vi "S2C_VLFT10_Proc_LaunchFornax.vi"(8 "Error In":errorcluster, 11 "Selection":string) -> (0 "Error Out":errorcluster, 3 "Version":string)   [LabVIEW 2015]
uses:
  Fornax/VIs/PolyDriver/Typedefs/ExternalCommCommand.ctl
  Fornax/VIs/S2C_FORNAX_Proc_Globals.vi
  Fornax/VIs/PolyDriver/S2C_FORNAX_Poly_CloseFornax.vi
  Fornax/VIs/PolyDriver/S2C_FORNAX_Poly_LaunchFornax.vi
  Fornax/VIs/PolyDriver/S2C_FORNAX_Poly_OpenSocket.vi
  Fornax/VIs/PolyDriver/S2C_FORNAX_Poly_ExternalCommCommand.vi
panel:
  out "Paired?":bool
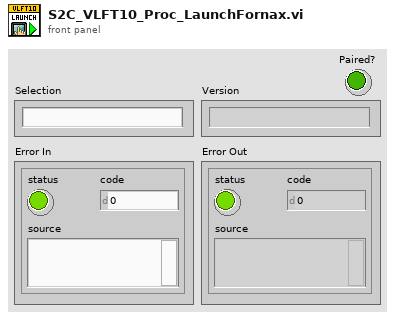
[diagram p1: front panel]
types:
  T1 = cluster{"Path":string, "Port":i32, "Version":u16}
  T2 = cluster{"Driver":string, "Command":string, "Return":string, "Parameters":string, "Timeout":dbl}
  T3 = typedef "ExternalCommCommand.ctl" = i16
  T4 = cluster{"Partition":string, "Message":string, "M_CommandOptions":string, "M_ControllerBoardId":string, "M_ClientId":string, "M_Command":T3}
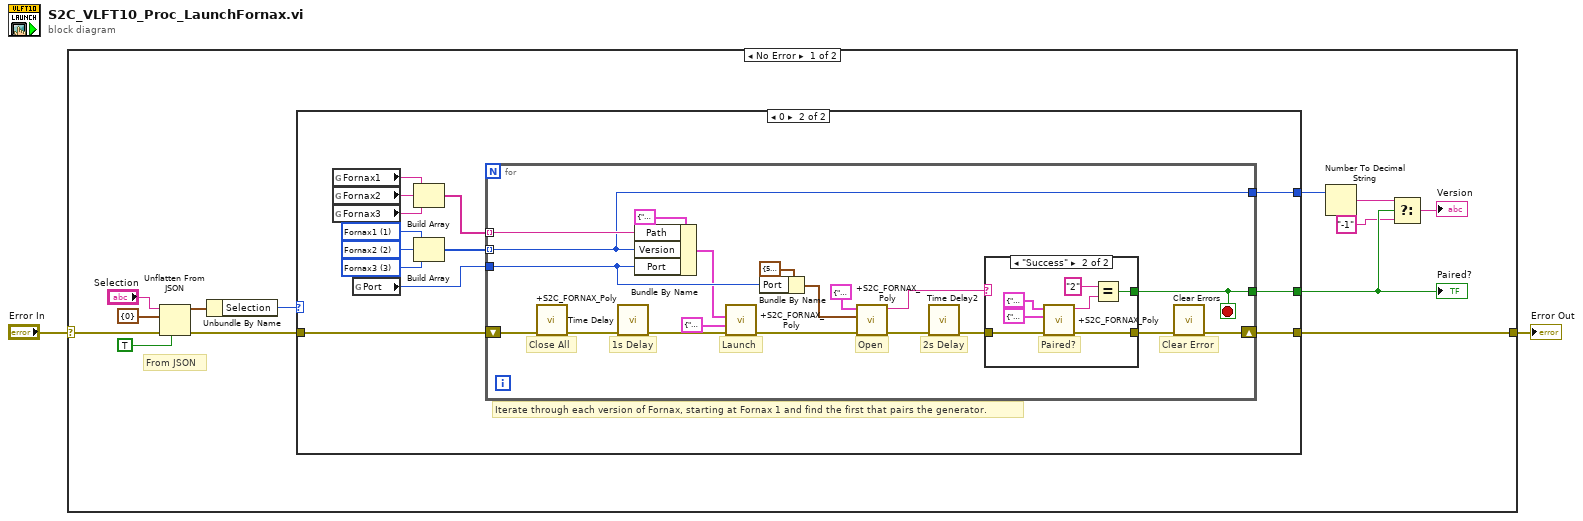
[diagram p0: block diagram]
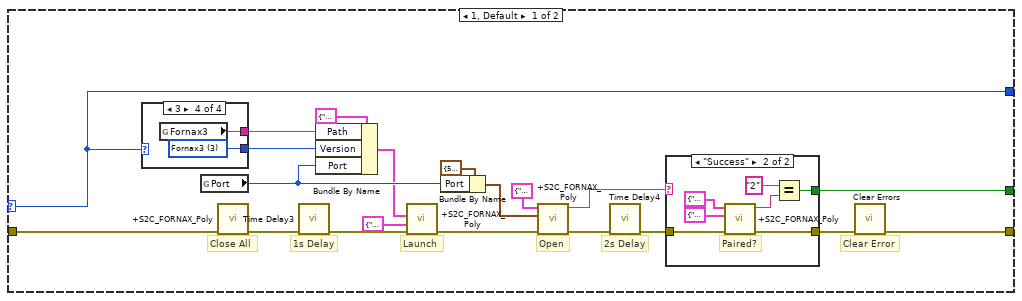
[diagram p2: hidden frame]
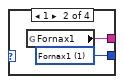
[diagram p4: hidden frame]
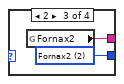
[diagram p5: hidden frame]
diagram:
  n1 = case shown="No Error" "Error In" {
    selector: "Error In" -> [w14 w90]
    tunnel: [w15 w90] -> w1
    frame No Error {
      # "From JSON"
      n2 = Unflatten From JSON(JSON string="Selection", type and defaults=cluster{"Selection":u16} {"Selection"=0}, default null elements? (F)=TRUE, error in (no error)=w14) -> (value=w9:cluster{"Selection":u16}, error out=w10:errorcluster)  [unwired: 3 in]
      n3 = Unbundle By Name(w9) -> ("Selection"=w8:u16)
      n4 = case shown="0" w8 {
        selector: w8 -> [w16 _]
        tunnel: [w34 w61] -> w15
        tunnel: [w33 w52] -> w5
        tunnel: w10 -> [w32 w51]
        tunnel: [w16 w50] -> w7
        frame 1, Default {
          # "Clear Error"
          # "2s Delay"
          # "1s Delay"
          # "Open"
          # "Launch"
          # "Close All"
          n5 = case shown="3" w16 {
            tunnel: [_ w37 w39 w41] -> w18
            tunnel: [_ w36 w38 w40] -> w17
            frame 0, Default {
            }
            frame 1 {
              w36 = u16 1 items=["Fornax1"=1, "Fornax2"=2, "Fornax3"=3] ("Version")
              n6 = global read "S2C_FORNAX_Proc_Globals.vi" "Fornax1"() -> (w37:string)
            }
            frame 2 {
              w38 = u16 2 items=["Fornax1"=1, "Fornax2"=2, "Fornax3"=3] ("Version")
              n7 = global read "S2C_FORNAX_Proc_Globals.vi" "Fornax2"() -> (w39:string)
            }
            frame 3 {
              w40 = u16 3 items=["Fornax1"=1, "Fornax2"=2, "Fornax3"=3] ("Version")
              n8 = global read "S2C_FORNAX_Proc_Globals.vi" "Fornax3"() -> (w41:string)
            }
          }
          n9 = global read "S2C_FORNAX_Proc_Globals.vi" "Port"() -> (w35:i32)
          n10 = call-poly "+S2C_FORNAX_Poly.vi"("Error In"=w32) -> ("Error Out"=w19:errorcluster)  [unwired: 9 in, 1 out]
          n11 = call "Time Delay3"("error in (no error)"=w19) -> ("error out"=w25:errorcluster)  [unwired: 10 in]
          n12 = Bundle By Name(cluster=T1 {"Path"="", "Port"=50000, "Version"=1} ("Open"), "Path"=w18, "Version"=w17, "Port"=w35) -> (w23:T1)
          n13 = call-poly "+S2C_FORNAX_Poly.vi"("Error In"=w25, "Open"=w23, "Settings"=T2 {"Driver"="Fornax", "Command"="Launch", "Return"="ErrorStatus", "Parameters"="", "Timeout"=10.0}) -> ("Error Out"=w31:errorcluster)  [unwired: 7 in, 1 out]
          n14 = Bundle By Name(cluster=cluster{"Port":i32} {"Port"=50000} ("Open"), "Port"=w35) -> (w29:cluster{"Port":i32})
          n15 = call-poly "+S2C_FORNAX_Poly.vi"("Error In"=w31, "Open"=w29, "Settings"=T2 {"Driver"="Fornax", "Command"="Open", "Return"="ErrorStatus", "Parameters"="", "Timeout"=20.0}) -> ("Error Out"=w22:errorcluster, "Response"=w27:string)  [unwired: 7 in]
          n16 = call "Time Delay4"("error in (no error)"=w22) -> ("error out"=w21:errorcluster)  [unwired: 10 in]
          n17 = case shown="\"Success\"" w27 {
            tunnel: w21 -> [w42 w49]
            tunnel: [w42 w45] -> w20
            tunnel: [_ w44] -> w33
            frame "Other", Default {
            }
            frame "Success" {
              # "Paired?"
              n18 = call-poly "+S2C_FORNAX_Poly.vi"("Error In"=w49, "ExternalCommCommand"=T4 {"Partition"="Default", "Message"="ExternalCommCommand", "M_CommandOptions"="", "M_ControllerBoardId"="", "M_ClientId"="", "M_Command"=5}, "Settings"=T2 {"Driver"="Fornax", "Command"="ExternalCommCommand", "Return"="M_PairingStatus", "Parameters"="", "Timeout"=10.0}) -> ("Error Out"=w45:errorcluster, "Response"=w47:string)  [unwired: 7 in]
              n19 = Equal?(x="2", y=w47) -> (x = y?=w44:bool)
            }
          }
          n20 = call <vilib>:"Clear Errors.vi"("error in (no error)"=w20) -> ("error out"=w34:errorcluster)  [unwired: 5 in, 1 out]
        }
        frame 0 {
          w55 = u16 3 items=["Fornax1"=1, "Fornax2"=2, "Fornax3"=3] ("Version")
          w57 = u16 2 items=["Fornax1"=1, "Fornax2"=2, "Fornax3"=3] ("Version")
          w56 = u16 1 items=["Fornax1"=1, "Fornax2"=2, "Fornax3"=3] ("Version")
          # "Iterate through each version of Fornax, starting at Fornax 1 and find the first that pairs the generator."
          n21 = global read "S2C_FORNAX_Proc_Globals.vi" "Fornax1"() -> (w59:string)
          n22 = global read "S2C_FORNAX_Proc_Globals.vi" "Fornax2"() -> (w60:string)
          n23 = global read "S2C_FORNAX_Proc_Globals.vi" "Fornax3"() -> (w58:string)
          n24 = global read "S2C_FORNAX_Proc_Globals.vi" "Port"() -> (w62:i32)
          n25 = Build Array(w59, w60, w58) -> (w54:string[])
          n26 = Build Array(w56, w57, w55) -> (w53:u16[])
          n27 = for {
            tunnel: w62 -> [w79]
            tunnel: w54 -> [w71] mode=indexing
            tunnel: w53 -> [w63] mode=indexing
            shift-right: [w67] -> w61
            shift-left: w51 -> [w64]
            tunnel: [w66] -> w52
            tunnel: [w63] -> w50
            stop <- w66 stop-if-true
            # "Clear Error"
            # "2s Delay"
            # "1s Delay"
            # "Open"
            # "Launch"
            # "Close All"
            n28 = call-poly "+S2C_FORNAX_Poly.vi"("Error In"=w64) -> ("Error Out"=w65:errorcluster)  [unwired: 9 in, 1 out]
            n29 = call "Time Delay"("error in (no error)"=w65) -> ("error out"=w74:errorcluster)  [unwired: 10 in]
            n30 = Bundle By Name(cluster=T1 {"Path"="", "Port"=50000, "Version"=1} ("Open"), "Path"=w71, "Version"=w63, "Port"=w79) -> (w72:T1)
            n31 = call-poly "+S2C_FORNAX_Poly.vi"("Error In"=w74, "Open"=w72, "Settings"=T2 {"Driver"="Fornax", "Command"="Launch", "Return"="ErrorStatus", "Parameters"="", "Timeout"=10.0}) -> ("Error Out"=w81:errorcluster)  [unwired: 7 in, 1 out]
            n32 = Bundle By Name(cluster=cluster{"Port":i32} {"Port"=50000} ("Open"), "Port"=w79) -> (w78:cluster{"Port":i32})
            n33 = call-poly "+S2C_FORNAX_Poly.vi"("Error In"=w81, "Open"=w78, "Settings"=T2 {"Driver"="Fornax", "Command"="Open", "Return"="ErrorStatus", "Parameters"="", "Timeout"=20.0}) -> ("Error Out"=w70:errorcluster, "Response"=w76:string)  [unwired: 7 in]
            n34 = call "Time Delay2"("error in (no error)"=w70) -> ("error out"=w69:errorcluster)  [unwired: 10 in]
            n35 = case shown="\"Success\"" w76 {
              tunnel: w69 -> [w82 w89]
              tunnel: [w82 w85] -> w68
              tunnel: [_ w84] -> w66
              frame "Other", Default {
              }
              frame "Success" {
                # "Paired?"
                n36 = call-poly "+S2C_FORNAX_Poly.vi"("Error In"=w89, "ExternalCommCommand"=T4 {"Partition"="Default", "Message"="ExternalCommCommand", "M_CommandOptions"="", "M_ControllerBoardId"="", "M_ClientId"="", "M_Command"=5}, "Settings"=T2 {"Driver"="Fornax", "Command"="ExternalCommCommand", "Return"="M_PairingStatus", "Parameters"="", "Timeout"=10.0}) -> ("Error Out"=w85:errorcluster, "Response"=w87:string)  [unwired: 7 in]
                n37 = Equal?(x="2", y=w87) -> (x = y?=w84:bool)
              }
            }
            n38 = call <vilib>:"Clear Errors.vi"("error in (no error)"=w68) -> ("error out"=w67:errorcluster)  [unwired: 5 in, 1 out]
          }
        }
      }
      "Paired?" <- w5
      n39 = Number To Decimal String(number=w7) -> (decimal integer string=w6:string)  [unwired: 1 in]
      n40 = Select(t=w6, s=w5, f="-1") -> (s? t:f=→"Version":string)
    }
    frame Error {
    }
  }
  "Error Out" <- w1
